vi "ETMF_ACP.vi"() -> ()   [LabVIEW 2019]
uses:
  <vilib>/Utility/error.llb/DialogType.ctl
  <vilib>/DAQmx/write.llb/DAQmx Write (Digital Bool 1Line 1Point).vi
  <vilib>/DAQmx/write.llb/DAQmx Write (Counter Frequency 1Chan 1Samp).vi
  <vilib>/DAQmx/miscellaneous.llb/DAQmx Fill In Error Info.vi
  <vilib>/DAQmx/create/channels.llb/DAQmx Create Channel (CO-Pulse Generation-Frequency).vi
  <vilib>/DAQmx/configure/timing.llb/DAQmx Timing (Implicit).vi
  <vilib>/addons/control/pid/pid.llb/PID (DBL).vi
  <vilib>/Utility/file.llb/Write Delimited Spreadsheet (string).vi
  <instrlib>/Agilent 34970/Agilent 34970.lvlib
  <resource>/objmgr/daqmx.rc
  <vilib>/addons/control/pid/NI_PID_pid.lvlib
  <instrlib>/Yokogawa WT200 Series/Yokogawa WT200 Series.lvlib
  <instrlib>/Agilent 681x Series/Agilent 681x Series.lvlib
panel:
  in  "Tab Control":T1(tab)
  in  "Ts":dbl=1.0
  out "Time":dbl=300.0 format="%<%H:%M:%S>t"
  in  "STOP":bool
  in  "Idenfier_Estufa":string="medsForno"
  in  "Estufa_ON":bool=TRUE
  in  "Frequency":dbl=1.0 format="%.6f"
  in  "PID gains":T2={"proportional gain (Kc)"=39.6, "integral time (Ti, min)"=14.617, "derivative time (Td, min)"=0.0} {"derivative time (Td, min)" format="%.3f"; "integral time (Ti, min)" format="%.3f"; "proportional gain (Kc)" format="%.6f"}
  out "Process variable and Setpoint":cluster{"initial PV":dbl, "SP:":dbl}(graph)
  out "MV":dbl(graph)
  in  "SP:":dbl(slide)=70.0 min=0.0 max=0.0 scale=25.0..70.0
  out "Temperature CH9 [degC]":dbl
  out "Temperature CH4 [degC]":dbl
  out "Iteration":i32
  out "Duty Cycle":sgl=0.1 min=0.1 max=99.9 format="%#_6f"
  out "PV":dbl
  in  "Tempo de integração (s)":u32=5 min=1 max=60 step=1
  out "Chart tensão numeric":cluster{"V(A)":dbl, "V(B)":dbl, "V(E)":dbl}(graph)={"V(A)"=0.0, "V(B)"=0.0, "V(E)"=228.25999450683594}
  out "Chart corrente numeric":cluster{"I(A)":dbl, "I(B)":dbl, "I(E)":dbl}(graph)={"I(A)"=0.0, "I(B)"=0.0, "I(E)"=0.14239999651908875}
  out "Chart potencia numeric":T3(graph)={"PC(A)"=0.0, "PC(B)"=7.200000254670158e-05, "PC(T)"=7.200000254670158e-05, "PL(A)"=0.0, "PL(B)"=0.0, "PL(T)"=0.0, "PC(E)"=1.0970638990402222, "PL(E)"=1.0099999904632568}
  in  "Realiza medição WT230":bool=TRUE
  in  "Medição contínua? WT230":bool=TRUE
  in  "Parâmetros serial":T4={"Serial VCC"="COM7", "timeout"=2, "baud rate"=600, "flow control"=0, "data bits"=8, "parity"=enum."None", "stop bits"=10, "termination char"=FALSE} {"stop bits" items=["1.0"=10, "1.5"=15, "2.0"=20]; "flow control" items=["None", "XON/XOFF", "RTS/CTS", "XON/XOFF & RTS/CTS", "DTR/DSR", "XON/XOFF & DTR/DSR"]}
  in  "Velocidade (RPM)":u16 min=1000 max=10000 step=100
  in  "Mensagem":T5(ring)=enum."Read power"
  in  "Limite de corrente":dbl min=0.0 max=0.4 step=0.01 format="%.4f"
  in  "Limite de tensão":dbl=30.0 min=0.0 max=30.0 step=0.5 format="%.4f"
  in  "Seta carga":bool
  in  "Enviar velocidade":bool
  in  "Envia mensagem":bool
  in  "Parar motor":bool
  out "Tradução":string
  out "Resposta":string
  in  "Liga Fonte":bool
  out "watt num cluster":T6
  out "Corrente de saída":dbl format="%.4f"
  out "Tensão de saída":dbl format="%.4f"
  out "t":dbl
  out "PL(T)":dbl
  out "PC(T)":dbl
  out "PC(E)":dbl
  out "PL(E)":dbl
  in  "Identifier_Watt":string="medsWatt"
  in  "Idenfier_Freio":string="medsFreio"
  in  "Manual":bool
  out "MV_I":dbl(graph)
  in  "PID gains MF":T2={"proportional gain (Kc)"=307.5977, "integral time (Ti, min)"=0.2636, "derivative time (Td, min)"=0.0} {"derivative time (Td, min)" format="%.3f"; "integral time (Ti, min)" format="%.3f"; "proportional gain (Kc)" format="%.6f"}
  out "Grafico MF ENS":cluster{"initial PV":dbl, "SP:":dbl}(graph)
  out "MV_MF":sgl=0.1 min=0.1 max=99.9 format="%#_6f"
  out "PV_MF":dbl
  in  "Ts MF":dbl=5.0
  in  "Automatic":bool
  in  "SP_MF":dbl(slide)=70.0 caption="SP:" min=0.0 max=0.0 scale=25.0..70.0
  in  "Ident_EnsTerMF":string="medsETMF"
  in  "Tab Control 2":enum32{"1-7", "8-15"}(tab)
  out "G. TP 1":cluster{dbl, "index":i32}(graph)
  out "TP 1":dbl
  out "TP 2":dbl
  out "G. TP 2":cluster{dbl, "index":i32}(graph)
  out "G. TP 3":cluster{dbl, "index":i32}(graph)
  out "TP 3":dbl
  out "G. TP 5":cluster{dbl, "index":i32}(graph)
  out "TP 5":dbl
  out "G. TP 6":cluster{dbl, "index":i32}(graph)
  out "TP 6":dbl
  out "G. TP 7":cluster{dbl, "index":i32}(graph)
  out "TP 7":dbl
  out "G. TP 8":cluster{dbl, "index":i32}(graph)
  out "TP 8":dbl
  out "G. TP 10":cluster{dbl, "index":i32}(graph)
  out "TP 10":dbl
  out "G. TP 11":cluster{dbl, "index":i32}(graph)
  out "TP 11":dbl
  out "G. TP 12":cluster{dbl, "index":i32}(graph)
  out "TP 12":dbl
  out "G. TP 13":cluster{dbl, "index":i32}(graph)
  out "TP 13":dbl
  out "G. TP 15":cluster{dbl, "index":i32}(graph)
  out "TP 15":dbl
  in  "Idenfier_Ens. Term.":string="medsETMA"
  out "Chart Temperatura":cluster{dbl, dbl, dbl, dbl, dbl, dbl}(graph)={21.505, 22.941, 24.092, 23.94, 23.972, 20.648}
  out "temperature num cluster":T7
  in  "Pulse Characteristic Value (%)":dbl=100.0 format="%#.4g"
  in  "Pulse Count":dbl=1.0 format="%#.4g"
  in  "Pulse Characteristic (0: Duty Cycle)":u16(ring) items=["Duty Cycle", "Pulse Width"]
  in  "Period (s)":dbl=10.0 format="%#.4g"
  in  "Output Frequency (60 Hz)":dbl=60.0 format="%#.4g"
  in  "Voltage Mode (0: Fix)":u16(ring) items=["Fixed", "Step", "Pulse", "List"]
  in  "Voltage Amplitude (1.0 V)":dbl=1.0 format="%#.4g"
  in  "Trigger Delay (s)":dbl=10.0 format="%#.5g"
  in  "Triggered Voltage Amplitude (V)":dbl=1.0 format="%#.4g"
  in  "Output Waveform Type (0: Sinusoid)":u16(ring) items=["Sinusoid", "Square", "Clipped Sinusoid", "User Specified"]
  in  "Peak Current Limit (13 A)":dbl=13.0 format="%#.4g"
  in  "RMS Current Limit (1 A)":dbl=1.0 format="%#.4g"
  in  "VISA resource name":refnum<visa-resource-name>
  out "CurMeas":T8
  out "PwrMeas":T9
  out "ACP_CUR":T10(graph)
  in  "Idenfier_Meas6812B":string="meds6812B"
  out "error out":errorcluster
  in  "Serial Configuration":T11={"Baud Rate"=9600, "Parity"=0, "Data Bits"=8} {"Data Bits" items=["7"=7, "8"=8]; "Parity" items=["None", "Odd", "Even", "Mark", "Space"]; "Baud Rate" items=["300"=300, "600"=600, "1200"=1200, "2400"=2400, "4800"=4800, "9600"=9600]}
  out "ACP_PWR":T12(graph)
  # "Controle de Temperatura da Estufa"
  # "Geral"
  # "Respostas do Sistema em Malha Fechada"
  # "Controles"
  # "Medidas"
  # "Freio"
  # "Wattímetro WT230 Yokogawa"
  # "Controles:"
  # "Controles"
  # "Medidas"
  # "Respostas temporais"
  # "Medidas"
  # "Inversor de Frequência"
  # "Controles"
  # "Comandos"
  # "Parâmetros Serial"
  # "Controle Automático do Ensaio de Estresse Térmico"
  # "Geral"
  # "Controles"
  # "Medidas"
  # "Temperaturas dos Termopares"
  # "Nome do arquivo:"
  # "Legenda:"
  # "TP 1: Termopar do Capacitor C011"
  # "TP 3: Termopar do Choke L001"
  # "TP 2: Termopar do Capacitor C009"
  # "TP 5: Termopar do Capacitor C006"
  # "TP 6: Termopar do Fusível F002"
  # "TP 7: Termopar do Conector CN204"
  # "TP 8: Termopar do CI SMPS IC 100"
  # "TP 10: Termopar do Indutor L100"
  # "TP 11: Termopar do Capacitor C112"
  # "TP 12: Termopar do Capacitor C504"
  # "TP 13: Termopar do Microcontrolador IC601"
  # "TP 15: Termopar do Dissipador"
  # "Temperaturas do Motor/Freio"
  # "Gráficos:"
  # "Configurações da Saída"
  # "Potências:"
  # "Trigger"
  # "Forma de Onda"
  # "Correntes:"
  # "Proteção contra Sobrecorrente"
  # "Comunicação"
  # "Fonte AC Programável - Agilent 6812B"
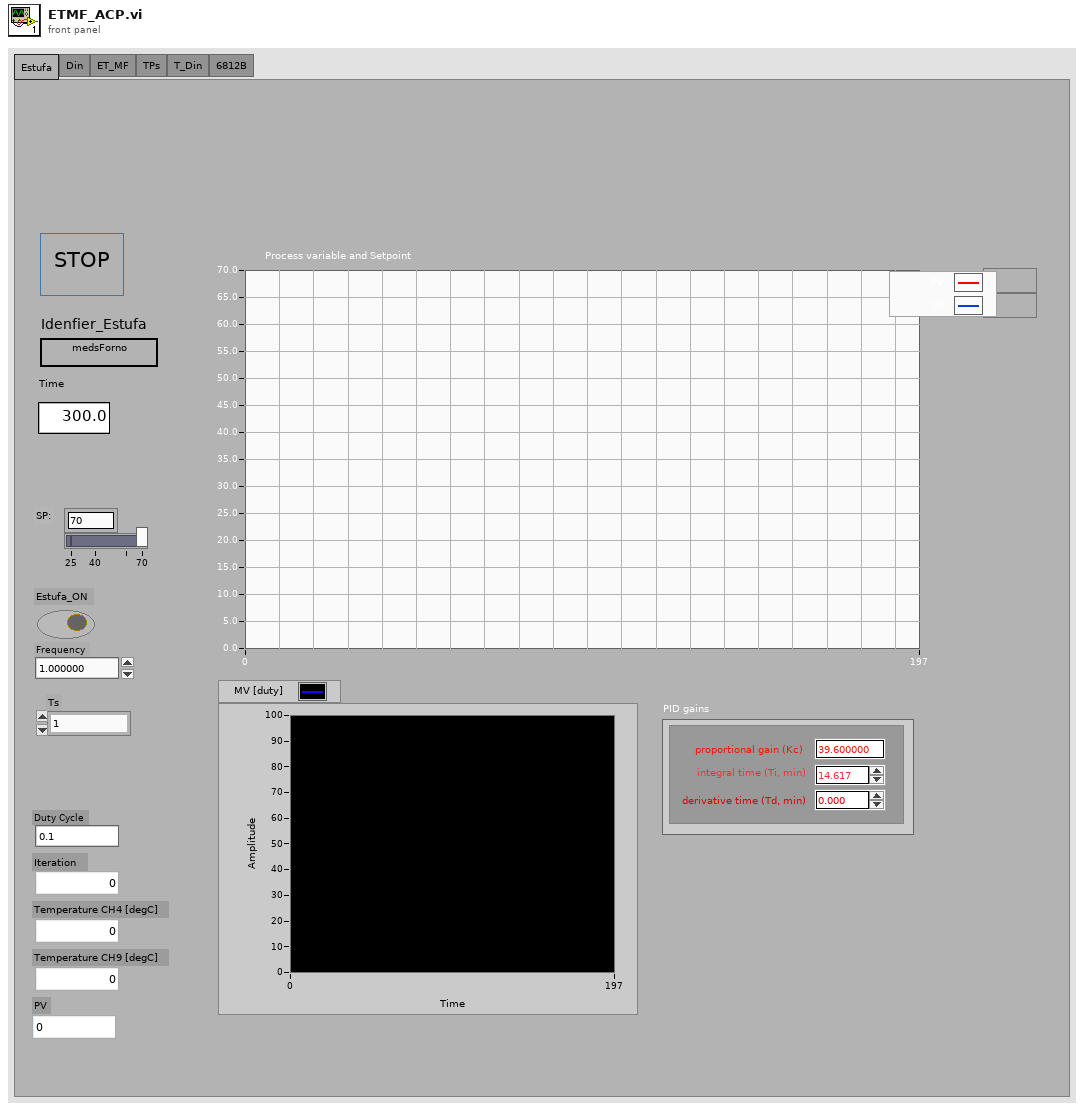
[diagram p1: front panel]
types:
  T1 = enum32{"Estufa", "Din", "ET_MF", "TPs", "T_Din", "6812B"}
  T2 = cluster{"proportional gain (Kc)":dbl, "integral time (Ti, min)":dbl, "derivative time (Td, min)":dbl}
  T3 = cluster{"PC(A)":dbl, "PC(B)":dbl, "PC(T)":dbl, "PL(A)":dbl, "PL(B)":dbl, "PL(T)":dbl, "PC(E)":dbl, "PL(E)":dbl}
  T4 = cluster{"Serial VCC":refnum<visa-resource-name>, "timeout":u32, "baud rate":u32, "flow control":u16, "data bits":u16, "parity":enum16{"None", "Odd", "Even", "Mark", "Space"}, "stop bits":u16, "termination char":bool}
  T5 = enum16{"Read set speed", "Read operation status", "Read power", "Read starting trials", "Read bus voltage", "Read temperature", "Read power limitation", "Read PWM mode", "Read PWM frequency", "Read real speed"}
  T6 = cluster{"V(A)":dbl, "I(A)":dbl, "V(B)":dbl, "I(B)":dbl, "PC(A)":dbl, "PC(B)":dbl, "PC(T)":dbl, "PL(T)":dbl, "PL(B)":dbl, "PL(A)":dbl, "V(E)":dbl, "PL(E)":dbl, "PC(E)":dbl, "I(E)":dbl, "t":dbl}
  T7 = cluster{"t1 freio":dbl, "t2 bobina":dbl, "t5 bobina":dbl, "t4 estator":dbl, "t3 estator":dbl, "t6 amb":dbl}
  T8 = cluster{"Peak Current":dbl, "DC Current":dbl, "AC RMS Current":dbl, "AC + DC RMS Cur":dbl}
  T9 = cluster{"Power Factor":dbl, "Reactive Power":dbl, "DC Power":dbl, "Real Power":dbl, "Apparent Power":dbl, "Total Power":dbl}
  T10 = cluster{"Peak Current":dbl, "AC RMS Current":dbl, "AC + DC RMS Current":dbl}
  T11 = cluster{"Baud Rate":u32, "Parity":u16, "Data Bits":u16}
  T12 = cluster{"Reactive Power":dbl, "Apparent Power":dbl, "Total Power":dbl}
  T13 = enum16{"Start Comm.", "End Comm.", "Wait", "Send Static Message", "Set Speed"}
  T14 = enum16{"Thermocouple", "Thermistor", "RTD", "4-Wire RTD", "Default (Last)"}
  T15 = enum8{"Enabled", "Disabled", "Disabled and Grayed Out"}
  T16 = cluster{"Peak Current":dbl, "DC Current":dbl, "AC RMS Current":dbl, "AC + DC RMS Current":dbl}
  T17 = cluster{"Peak Current":dbl, "AC RMS Current":dbl, "AC + DC RMS Cur":dbl}
  T18 = typedef "DialogType.ctl" = u16
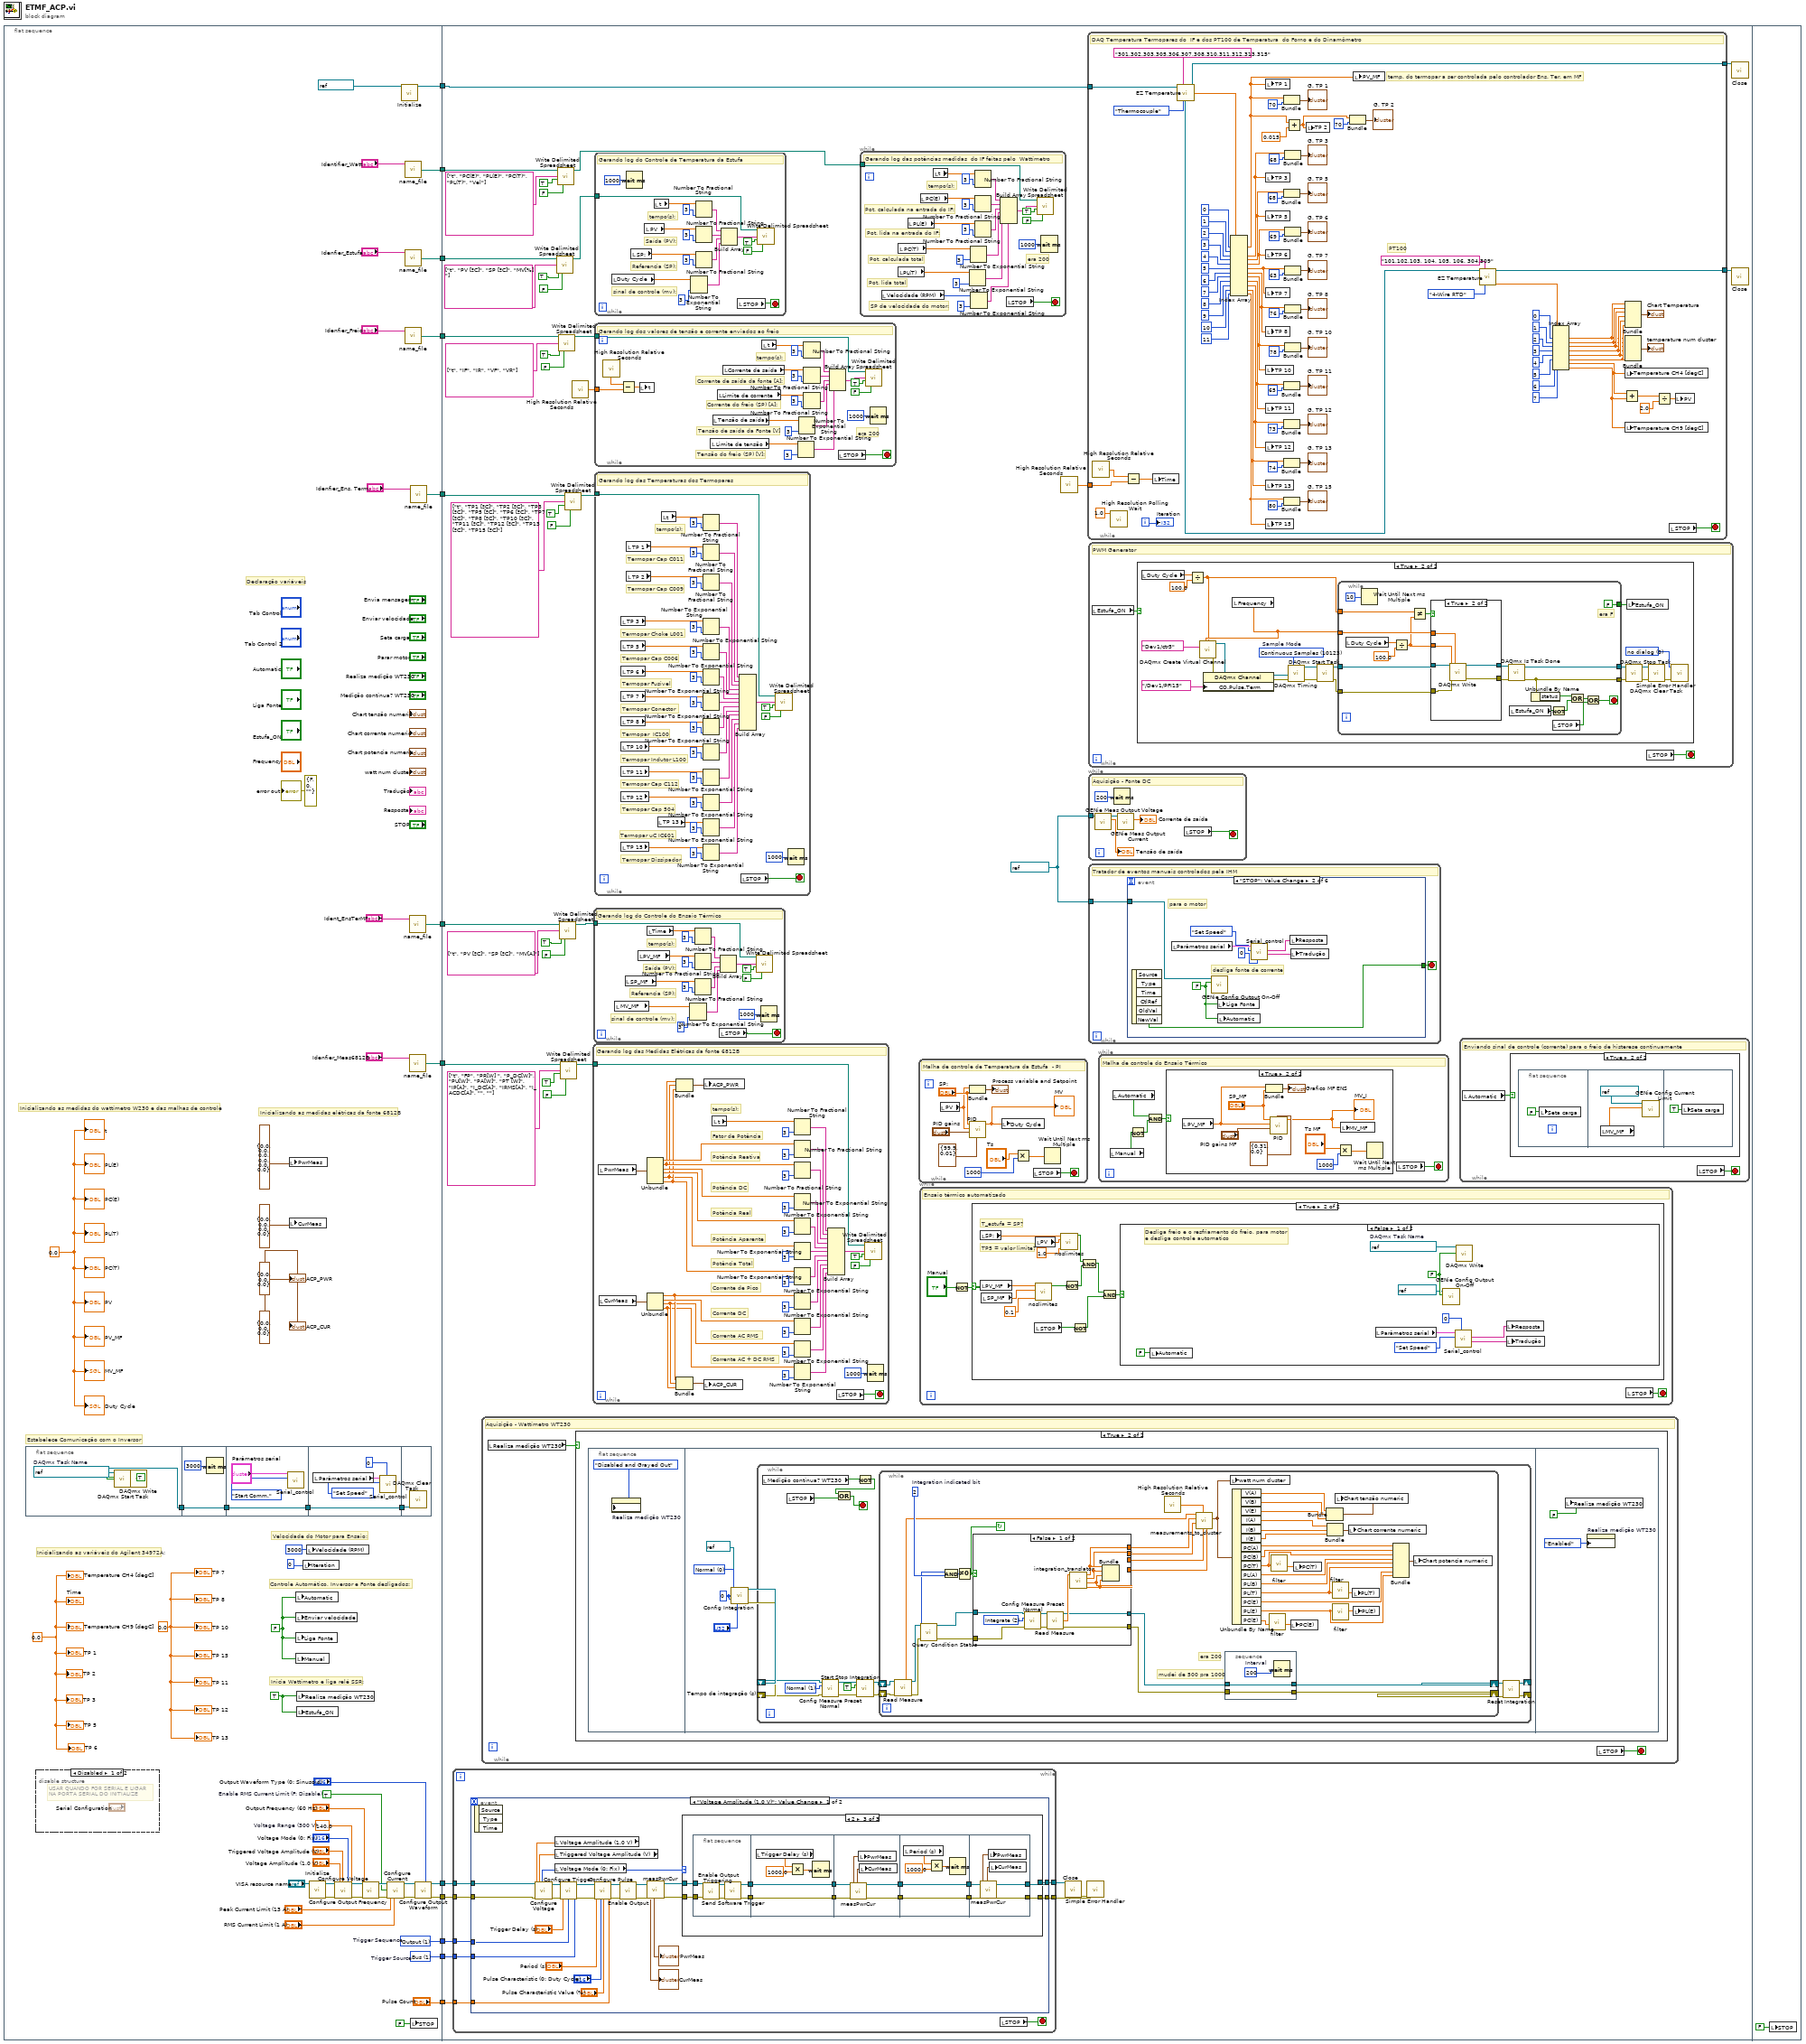
[diagram p0: block diagram]
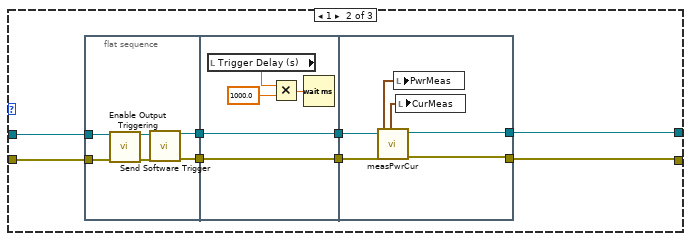
[diagram p4: hidden frame]
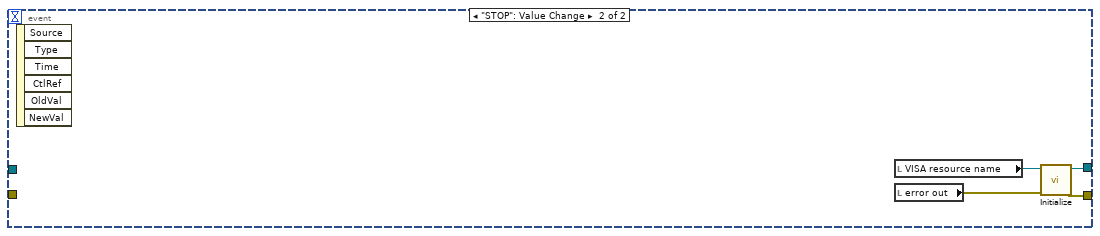
[diagram p5: hidden frame]
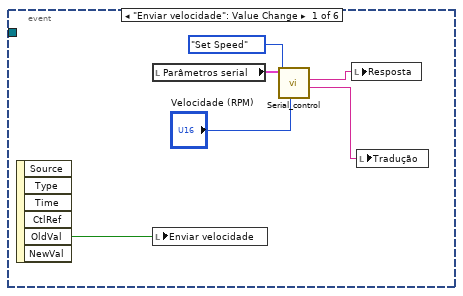
[diagram p7: hidden frame]
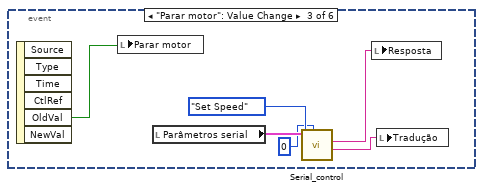
[diagram p8: hidden frame]
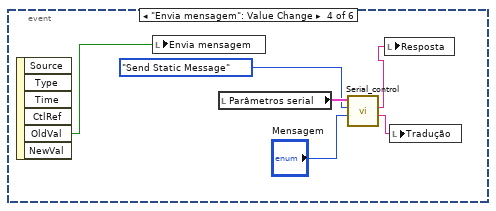
[diagram p9: hidden frame]
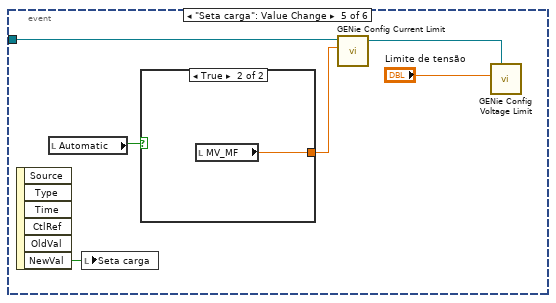
[diagram p10: hidden frame]
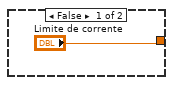
[diagram p11: hidden frame]
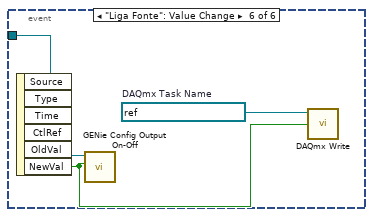
[diagram p12: hidden frame]
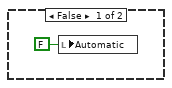
[diagram p14: hidden frame]
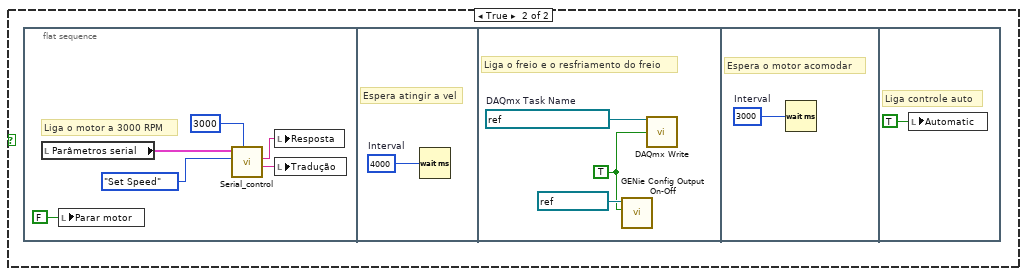
[diagram p15: hidden frame]
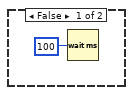
[diagram p16: hidden frame]
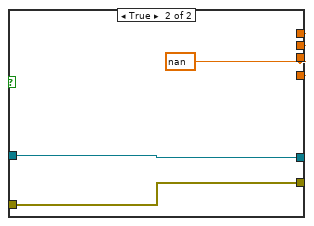
[diagram p17: hidden frame]
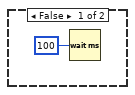
[diagram p18: hidden frame]
diagram:
  n1 = flat-sequence {
    tunnel: [w64] -> w12
    tunnel: [w63] -> w11
    tunnel: [w59] -> w10
    tunnel: [w57] -> w9
    tunnel: [w55] -> w8
    tunnel: [w52] -> w7
    tunnel: [w48] -> w6
    tunnel: [w25] -> w5
    tunnel: [w24] -> w4
    tunnel: [w22] -> w3
    tunnel: [w23] -> w2
    tunnel: ["Pulse Count"] -> w1
    tunnel: w12 -> [w98]
    tunnel: w11 -> [w118]
    tunnel: w10 -> [w117]
    tunnel: w9 -> [w112]
    tunnel: w8 -> [w103]
    tunnel: w7 -> [w94]
    tunnel: w6 -> [w91]
    tunnel: w5 -> [w84]
    tunnel: w4 -> [w83]
    tunnel: w3 -> [w82]
    tunnel: w2 -> [w81]
    tunnel: w1 -> [w80]
    frame #0 {
      w23 = 1 items=["Immediate", "Bus", "External", "Phase", "Trigger Out"]  # Trigger Source
      w22 = 1 items=["Output"=1, "Synchronous Source"=2, "Measurement"=3]  # Trigger Sequence
      w27 = TRUE  # Enable RMS Current Limit (F: Disable)
      w26 = 140.0  # Voltage Range (300 V)
      w45 = 0.0 ("Temperature 1")
      w46 = 0.0 ("PC(E)")
      w49 = FALSE ("Automatic")
      w50 = TRUE ("Realiza medição WT230")
      w54 = 0.0 ("Temperature 1")
      # "Estabelece Comunicação com o Inversor"
      # "Inicializando as variáveis do Agilent 34972A:"
      # "Inicializando as medidas do wattímetro W230 e das malhas de controle"
      # "Inicializando as medidas elétricas da fonte 6812B"
      # "Inicia Wattímetro e liga relé SSR:"
      # "Controle Automático, Inversor e Fonte desligados:"
      # "Velocidade do Motor para Ensaio:"
      # "Declaração variáveis"
      n2 = flat-sequence {
        tunnel: [w66] -> w16
        tunnel: w16 -> [w69]
        tunnel: [w69] -> w15
        tunnel: w15 -> [w71]
        tunnel: [w71] -> w14
        tunnel: w14 -> [w74]
        tunnel: [w74] -> w13
        tunnel: w13 -> [w78]
        frame #0 {
          w67 = refnum<k21> "alimentacao_inversor"  # DAQmx Task Name
          n3 = call <vilib>:"DAQmx Start Task.vi"("task/channels in"=w67) -> ("task out"=w66:refnum<k21>)  [unwired: 13 in, 1 out]
          n4 = call-poly <vilib>:"DAQmx Write.vi"("task/channels in"=w66, "data"=TRUE) -> ()  [unwired: 11 in, 3 out]
        }
        frame #1 {
          n5 = Wait (ms)(milliseconds to wait=u32 3000) -> ()  [unwired: 1 out]
        }
        frame #2 {
          n6 = call "Serial_control.vi"("Função"=T13."Start Comm.", "comm cluster"="Parâmetros serial") -> ()  [unwired: 3 in, 4 out]
        }
        frame #3 {
          n7 = local read "Parâmetros serial"() -> (w76:T4)
          n8 = call "Serial_control.vi"("Enviar número"=u16 0, "Função"=T13."Set Speed", "comm cluster"=w76) -> ()  [unwired: 2 in, 4 out]
        }
        frame #4 {
          n9 = call <vilib>:"DAQmx Clear Task.vi"("task in"=w78) -> ()  [unwired: 14 in, 1 out]
        }
      }
      n10 = disable-structure shown="Disabled" {
        frame Disabled {
          # "USAR QUANDO FOR SERIAL E LIGAR \nNA PORTA SERIAL DO INITIALIZE"
        }
        frame Enabled {
        }
      }
      n11 = local write "PwrMeas"(T9 {"Power Factor"=0.0, "Reactive Power"=0.0, "DC Power"=0.0, "Real Power"=0.0, "Apparent Power"=0.0, "Total Power"=0.0} ("PwrMeas")) -> ()
      n12 = local write "CurMeas"(T8 {"Peak Current"=0.0, "DC Current"=0.0, "AC RMS Current"=0.0, "AC + DC RMS Cur"=0.0} ("CurMeas")) -> ()
      n13 = local write "Automatic"(w49) -> ()
      n14 = local write "Enviar velocidade"(w49) -> ()
      n15 = local write "Liga Fonte"(w49) -> ()
      n16 = local write "Manual"(w49) -> ()
      n17 = local write "Realiza medição WT230"(w50) -> ()
      n18 = local write "Estufa_ON"(w50) -> ()
      n19 = local write "Iteration"(0 ("Iteration")) -> ()
      n20 = local write "Velocidade (RPM)"(u16 3000 ("Velocidade (RPM)")) -> ()
      n21 = call <instrlib>:"Initialize.vi"("VISA resource name"="VISA resource name") -> ("error out"=w39:errorcluster)  [unwired: 9 in, 1 out]
      n22 = call <instrlib>:"Configure Voltage.vi"("VISA resource name"="VISA resource name", "Triggered Voltage Amplitude (1.0 V)"="Triggered Voltage Amplitude (V)", "Voltage Range (300 V)"=w26, "Voltage Amplitude (1.0 V)"="Voltage Amplitude (1.0 V)", "Voltage Mode (0: Fix)"="Voltage Mode (0: Fix)", "error in (no error)"=w39) -> ("VISA resource name out"=w31:refnum<visa-resource-name>, "error out"=w30:errorcluster)  [unwired: 8 in]
      n23 = call <instrlib>:"Configure Output Frequency.vi"("VISA resource name"=w31, "Output Frequency (60 Hz)"="Output Frequency (60 Hz)", "error in (no error)"=w30) -> ("VISA resource name out"=w41:refnum<visa-resource-name>, "error out"=w42:errorcluster)  [unwired: 11 in]
      n24 = call <instrlib>:"Configure Current.vi"("VISA resource name"=w41, "Enable RMS Current Limit (F: Disable)"=w27, "RMS Current Limit (1 A)"="RMS Current Limit (1 A)", "error in (no error)"=w42, "Peak Current Limit (13 A)"="Peak Current Limit (13 A)") -> ("VISA resource name out"=w29:refnum<visa-resource-name>, "error out"=w28:errorcluster)  [unwired: 9 in]
      n25 = call <instrlib>:"Initialize.vi"("VISA Resource Name"=refnum<visa-resource-name> "Agilent" ("VISA AGILENT")) -> ("VISA Resource Name Out"=w64:refnum<visa-resource-name>)  [unwired: 13 in, 1 out]
      n26 = call "name_file.vi"("Identifier"="Identifier_Watt") -> ("appended path"=w59:path)  [unwired: 2 in]
      n27 = call "name_file.vi"("Identifier"="Idenfier_Estufa") -> ("appended path"=w63:path)  [unwired: 2 in]
      n28 = call "name_file.vi"("Identifier"="Idenfier_Freio") -> ("appended path"=w57:path)  [unwired: 2 in]
      n29 = call "name_file.vi"("Identifier"="Ident_EnsTerMF") -> ("appended path"=w52:path)  [unwired: 2 in]
      n30 = call "name_file.vi"("Identifier"="Idenfier_Meas6812B") -> ("appended path"=w48:path)  [unwired: 2 in]
      n31 = call "name_file.vi"("Identifier"="Idenfier_Ens. Term.") -> ("appended path"=w55:path)  [unwired: 2 in]
      n32 = local write "STOP"(FALSE ("STOP")) -> ()
      n33 = call <instrlib>:"Configure Output Waveform.vi"("VISA resource name"=w29, "Output Waveform Type (0: Sinusoid)"="Output Waveform Type (0: Sinusoid)", "error in (no error)"=w28) -> ("VISA resource name out"=w25:refnum<visa-resource-name>, "error out"=w24:errorcluster)  [unwired: 11 in]
      "Temperature CH4 [degC]" <- w54
      "Temperature CH9 [degC]" <- w54
      "Time" <- w54
      "Duty Cycle" <- w46
      "PV" <- w46
      "PC(T)" <- w46
      "PL(T)" <- w46
      "PC(E)" <- w46
      "t" <- w46
      "PL(E)" <- w46
      "TP 1" <- w54
      "TP 2" <- w54
      "TP 3" <- w54
      "TP 5" <- w54
      "TP 6" <- w54
      "TP 7" <- w45
      "TP 8" <- w45
      "TP 10" <- w45
      "TP 11" <- w45
      "TP 12" <- w45
      "TP 13" <- w45
      "TP 15" <- w45
      "MV_MF" <- w46
      "PV_MF" <- w46
      "error out" <- errorcluster {"status"=FALSE, "code"=0, "source"=""} ("error out")
      "ACP_CUR" <- T10 {"Peak Current"=0.0, "AC RMS Current"=0.0, "AC + DC RMS Current"=0.0} ("ACP_CUR")
      "ACP_PWR" <- T12 {"Reactive Power"=0.0, "Apparent Power"=0.0, "Total Power"=0.0} ("ACP_PWR")
    }
    frame #1 {
      w92 = refnum<visa-resource-name> "Lambda" ("VISA name")
      n34 = while {
        tunnel: w84 -> [w130]
        tunnel: w83 -> [w129]
        tunnel: [w123] -> w86
        tunnel: [w124] -> w85
        tunnel: w81 -> [w127]
        tunnel: w82 -> [w126]
        tunnel: w80 -> [w125]
        stop <- w128 stop-if-true
        n35 = event shown="[0] \"Voltage Amplitude (1.0 V)\": Value Change" {
          selector: _ -> [_ _]
          dyn-events: _ -> [_ _]
          timeout: _ -> [_ _]
          tunnel: w130 -> [w154 _]
          tunnel: w129 -> [w153 _]
          tunnel: w127 -> [w143 _]
          tunnel: w126 -> [w142 _]
          tunnel: w125 -> [w137 _]
          tunnel: [w135 w225] -> w124
          tunnel: [w134 w226] -> w123
          event "Voltage Amplitude (1.0 V)": Value Change {
            n36 = event-data() -> ()  [unwired: 1 in, 3 out]
            n37 = local read "Voltage Amplitude (1.0 V)"() -> (w152:dbl)
            n38 = local read "Triggered Voltage Amplitude (V)"() -> (w136:dbl)
            n39 = local read "Voltage Mode (0: Fix)"() -> (w133:u16)
            n40 = call <instrlib>:"Configure Voltage.vi"("VISA resource name"=w154, "Triggered Voltage Amplitude (1.0 V)"=w136, "Voltage Amplitude (1.0 V)"=w152, "Voltage Mode (0: Fix)"=w133, "error in (no error)"=w153) -> ("VISA resource name out"=w149:refnum<visa-resource-name>, "error out"=w148:errorcluster)  [unwired: 9 in]
            n41 = call <instrlib>:"Configure Trigger.vi"("VISA resource name"=w149, "Trigger Sequence (1: Output 1)"=w143, "Trigger Source (0: Immediate)"=w142, "error in (no error)"=w148, "Trigger Delay (0 s)"="Trigger Delay (s)") -> ("VISA resource name out"=w150:refnum<visa-resource-name>, "error out"=w151:errorcluster)  [unwired: 9 in]
            n42 = call <instrlib>:"Configure Pulse.vi"("VISA resource name"=w150, "Pulse Count (1)"=w137, "Period (0.0333 s)"="Period (s)", "error in (no error)"=w151, "Pulse Characteristic (0: Duty Cycle)"="Pulse Characteristic (0: Duty Cycle)", "Pulse Characteristic Value (50)"="Pulse Characteristic Value (%)") -> ("VISA resource name out"=w147:refnum<visa-resource-name>, "error out"=w146:errorcluster)  [unwired: 8 in]
            n43 = call <instrlib>:"Enable Output.vi"("VISA resource name"=w147, "error in (no error)"=w146) -> ("VISA resource name out"=w156:refnum<visa-resource-name>, "error out"=w155:errorcluster)  [unwired: 12 in]
            n44 = call "measPwrCur.vi"("VISA resource name"=w156, "error in (no error)"=w155) -> ("PwrMeas"=→"PwrMeas":T9, "CurMeas"=→"CurMeas":T16, "VISA resource name out"=w145:refnum<visa-resource-name>, "error out"=w144:errorcluster)  [unwired: 3 in]
            n45 = case shown="2" w133 {
              tunnel: w145 -> [w158 w166 w189]
              tunnel: w144 -> [w157 w165 w188]
              tunnel: [w157 w160 w184] -> w135
              tunnel: [w158 w159 w185] -> w134
              frame 0, Default {
              }
              frame 1 {
                n46 = flat-sequence {
                  tunnel: w166 -> [w170]
                  tunnel: w165 -> [w169]
                  tunnel: [w168] -> w163
                  tunnel: [w167] -> w161
                  tunnel: [w177] -> w164
                  tunnel: w163 -> [w177]
                  tunnel: [w176] -> w162
                  tunnel: w161 -> [w176]
                  tunnel: w164 -> [w181]
                  tunnel: w162 -> [w178]
                  tunnel: [w179] -> w160
                  tunnel: [w180] -> w159
                  frame #0 {
                    n47 = call <instrlib>:"Enable Output Triggering.vi"("VISA resource name"=w170, "error in (no error)"=w169) -> ("VISA resource name out"=w171:refnum<visa-resource-name>, "error out"=w172:errorcluster)  [unwired: 12 in]
                    n48 = call <instrlib>:"Send Software Trigger.vi"("VISA resource name"=w171, "error in (no error)"=w172) -> ("VISA resource name out"=w168:refnum<visa-resource-name>, "error out"=w167:errorcluster)  [unwired: 12 in]
                  }
                  frame #1 {
                    n49 = local read "Trigger Delay (s)"() -> (w175:dbl)
                    n50 = Multiply(x=w175, y=1000.0) -> (x*y=w173:dbl)
                    n51 = Wait (ms)(milliseconds to wait=w173) -> ()  [unwired: 1 out]
                  }
                  frame #2 {
                    n52 = call "measPwrCur.vi"("VISA resource name"=w181, "error in (no error)"=w178) -> ("PwrMeas"=w182:T9, "CurMeas"=w183:T16, "VISA resource name out"=w180:refnum<visa-resource-name>, "error out"=w179:errorcluster)  [unwired: 3 in]
                    n53 = local write "PwrMeas"(w182) -> ()
                    n54 = local write "CurMeas"(w183) -> ()
                  }
                }
              }
              frame 2 {
                n55 = flat-sequence {
                  tunnel: [w199] -> w195
                  tunnel: [w198] -> w194
                  tunnel: w189 -> [w197]
                  tunnel: w188 -> [w196]
                  tunnel: [w206] -> w193
                  tunnel: w195 -> [w206]
                  tunnel: [w205] -> w192
                  tunnel: w194 -> [w205]
                  tunnel: w193 -> [w212]
                  tunnel: w192 -> [w211]
                  tunnel: [w210] -> w191
                  tunnel: [w209] -> w190
                  tunnel: w191 -> [w213]
                  tunnel: w190 -> [w214]
                  tunnel: [w214] -> w187
                  tunnel: [w213] -> w186
                  tunnel: w187 -> [w222]
                  tunnel: w186 -> [w221]
                  tunnel: [w220] -> w185
                  tunnel: [w219] -> w184
                  frame #0 {
                    n56 = call <instrlib>:"Enable Output Triggering.vi"("VISA resource name"=w197, "error in (no error)"=w196) -> ("VISA resource name out"=w200:refnum<visa-resource-name>, "error out"=w201:errorcluster)  [unwired: 12 in]
                    n57 = call <instrlib>:"Send Software Trigger.vi"("VISA resource name"=w200, "error in (no error)"=w201) -> ("VISA resource name out"=w199:refnum<visa-resource-name>, "error out"=w198:errorcluster)  [unwired: 12 in]
                  }
                  frame #1 {
                    n58 = local read "Trigger Delay (s)"() -> (w204:dbl)
                    n59 = Multiply(x=w204, y=1000.0) -> (x*y=w202:dbl)
                    n60 = Wait (ms)(milliseconds to wait=w202) -> ()  [unwired: 1 out]
                  }
                  frame #2 {
                    n61 = call "measPwrCur.vi"("VISA resource name"=w212, "error in (no error)"=w211) -> ("PwrMeas"=w207:T9, "CurMeas"=w208:T16, "VISA resource name out"=w209:refnum<visa-resource-name>, "error out"=w210:errorcluster)  [unwired: 3 in]
                    n62 = local write "PwrMeas"(w207) -> ()
                    n63 = local write "CurMeas"(w208) -> ()
                  }
                  frame #3 {
                    n64 = local read "Period (s)"() -> (w215:dbl)
                    n65 = Multiply(x=w215, y=1000.0) -> (x*y=w217:dbl)
                    n66 = Wait (ms)(milliseconds to wait=w217) -> ()  [unwired: 1 out]
                  }
                  frame #4 {
                    n67 = call "measPwrCur.vi"("VISA resource name"=w222, "error in (no error)"=w221) -> ("PwrMeas"=w223:T9, "CurMeas"=w218:T16, "VISA resource name out"=w220:refnum<visa-resource-name>, "error out"=w219:errorcluster)  [unwired: 3 in]
                    n68 = local write "PwrMeas"(w223) -> ()
                    n69 = local write "CurMeas"(w218) -> ()
                  }
                }
              }
            }
          }
          event "STOP": Value Change {
            n70 = event-data() -> ()  [unwired: 1 in, 6 out]
            n71 = local read "VISA resource name"() -> (w227:refnum<visa-resource-name>)
            n72 = local read "error out"() -> (w224:errorcluster)
            n73 = call <instrlib>:"Initialize.vi"("error in (no error)"=w224, "VISA resource name"=w227) -> ("error out"=w225:errorcluster, "VISA resource name out"=w226:refnum<visa-resource-name>)  [unwired: 8 in]
          }
        }
        n74 = local read "STOP"() -> (w128:bool)
      }
      n75 = while {
        stop <- w570 stop-if-true
        # "Aquisição - Wattímetro WT230"
        n76 = local read "Realiza medição WT230"() -> (w571:bool)
        n77 = case shown="True" w571 {
          frame False {
            n78 = Wait (ms)(milliseconds to wait=u32 100) -> ()  [unwired: 1 out]
          }
          frame True {
            n79 = flat-sequence {
              frame #0 {
                n80 = property on="Realiza medição WT230" class="Bool (strict)"("DisabledEnum"=T15."Disabled and Grayed Out" ("Disabled")) -> ()  [unwired: 2 in, 2 out]
              }
              frame #1 {
                w576 = u16 0 items=["Normal", "Continuous"] ("Integ Mode (0: Normal)")
                w577 = u32 0 ("Hour (0)")
                n81 = call <instrlib>:"Config Integration.vi"("VISA resource name"=refnum<visa-resource-name> "WT", "Integ Mode (0: Normal)"=w576, "Hour (0)"=w577, "Minute (0)"=w577, "Second (0)"="Tempo de integração (s)") -> ("VISA resource name out"=w579:refnum<visa-resource-name>, "error out"=w578:errorcluster)  [unwired: 9 in]
                n82 = while {
                  shift-right: [w583] -> _
                  shift-left: w579 -> [w581]
                  shift-right: [w582] -> _
                  shift-left: w578 -> [w580]
                  stop <- w584 stop-if-true
                  w590 = u16 1 items=["Clear", "Normal", "Integrate"] ("Preset Pattern (0: Clear)")
                  n83 = local read "Medição contínua? WT230"() -> (w586:bool)
                  n84 = local read "STOP"() -> (w587:bool)
                  n85 = call <instrlib>:"Config Measure Preset Normal.vi"("VISA resource name"=w581, "Preset Pattern (0: Clear)"=w590, "error in (no error)"=w580) -> ("VISA resource name out"=w592:refnum<visa-resource-name>, "error out"=w591:errorcluster)  [unwired: 11 in]
                  n86 = call <instrlib>:"Start Stop Integration.vi"("VISA resource name"=w592, "Start/Stop (F: Stop)"=TRUE, "error in (no error)"=w591) -> ("VISA resource name out"=w595:refnum<visa-resource-name>, "error out"=w594:errorcluster)  [unwired: 11 in]
                  n87 = Not(x=w586) -> (.not. x?=w585:bool)
                  n88 = Or(x=w585, y=w587) -> (x .or. y?=w584:bool)
                  n89 = while {
                    shift-left: w595 -> [w635]
                    shift-right: [w623] -> w589
                    shift-left: w594 -> [w632]
                    shift-right: [w621] -> w588
                    stop <- w631 continue-if-true
                    w638 = u16 2  # Integration indicated bit
                    # "era 200"
                    # "mudei de 500 pra 1000"
                    n90 = call <instrlib>:"Read Measure.vi"("VISA resource name"=w635, "error in (no error)"=w632) -> ("VISA resource name out"=w634:refnum<visa-resource-name>, "Measure Value"=w625:sgl[], "error out"=w633:errorcluster)  [unwired: 10 in, 1 out]
                    n91 = call <instrlib>:"Query Condition Status.vi"("VISA resource name"=w634, "error in (no error)"=w633) -> ("VISA resource name out"=w620:refnum<visa-resource-name>, "Condition"=w636:u16, "error out"=w619:errorcluster)  [unwired: 11 in]
                    n92 = And(x=w636, y=w638) -> (x .and. y?=w637:u16)
                    n93 = Not Equal To 0?(x=w637) -> (x != 0?=w631:bool)
                    n94 = case shown="False" w631 {
                      tunnel: [w649 w656] -> w630
                      tunnel: [w648 w656] -> w629
                      tunnel: [w647 w656] -> w628
                      tunnel: [w646 w656] -> w627
                      tunnel: [w645 w655] -> w624
                      tunnel: [w644 w654] -> w622
                      tunnel: w620 -> [w643 w655]
                      tunnel: w619 -> [w642 w654]
                      frame False {
                        w650 = u16 2 items=["Clear", "Normal", "Integrate"] ("Preset Pattern (0: Clear)")
                        n95 = call <instrlib>:"Config Measure Preset Normal.vi"("VISA resource name"=w643, "Preset Pattern (0: Clear)"=w650, "error in (no error)"=w642) -> ("VISA resource name out"=w653:refnum<visa-resource-name>, "error out"=w652:errorcluster)  [unwired: 11 in]
                        n96 = call <instrlib>:"Read Measure.vi"("VISA resource name"=w653, "error in (no error)"=w652) -> ("VISA resource name out"=w645:refnum<visa-resource-name>, "Measure Value"=w651:sgl[], "error out"=w644:errorcluster)  [unwired: 10 in, 1 out]
                        n97 = call "integration_translator.vi"("Valores integração"=w651) -> ("PI(E)"=w646:sgl, "PI(T)"=w647:sgl, "PI(B)"=w648:sgl, "PI(A)"=w649:sgl)  [unwired: 7 in]
                        n98 = Bundle("PI(A)"=w649, "PI(B)"=w648, "PI(T)"=w647, "PI(E)"=w646) -> ()  [unwired: 1 in, 1 out]
                      }
                      frame True {
                        w656 = nan
                      }
                    }
                    n99 = call <vilib>:"High Resolution Relative Seconds.vi"() -> ("relative seconds"=w626:dbl)
                    n100 = call "measurements_to_cluster.vi"("PI(E)"=w627, "PI(T)"=w628, "relative seconds"=w626, "PI(B)"=w629, "PI(A)"=w630, "Measure Value"=w625) -> ("watt cluster"=w618:T6)  [unwired: 4 in, 1 out]
                    n101 = stacked-sequence {
                      tunnel: w624 -> [w640]
                      tunnel: [w640] -> w623
                      tunnel: w622 -> [w639]
                      tunnel: [w639] -> w621
                      frame #0 {
                        w641 = u32 200  # Interval
                        n102 = Wait (ms)(milliseconds to wait=w641) -> ()  [unwired: 1 out]
                      }
                    }
                    n103 = local write "watt num cluster"(w618) -> ()
                    n104 = Unbundle By Name(w618) -> ("V(A)"=w613:dbl, "V(B)"=w612:dbl, "V(E)"=w611:dbl, "I(A)"=w610:dbl, "I(B)"=w609:dbl, "I(E)"=w608:dbl, "PC(A)"=w607:dbl, "PC(B)"=w606:dbl, "PC(T)"=w605:dbl, "PL(A)"=w603:dbl, "PL(B)"=w602:dbl, "PL(T)"=w601:dbl, "PC(E)"=w600:dbl, "PL(E)"=w599:dbl, "PC(E)"=w597:dbl)
                    n105 = call "filter.vi"("input"=w597) -> ("output"=w596:dbl)  [unwired: 10 in]
                    n106 = call "filter.vi"("input"=w605) -> ("output"=w604:dbl)  [unwired: 10 in]
                    n107 = local write "PC(E)"(w596) -> ()
                    n108 = local write "PC(T)"(w604) -> ()
                    n109 = Bundle("V(A)"=w613, "V(B)"=w612, "V(E)"=w611) -> (w617:cluster{"V(A)":dbl, "V(B)":dbl, "V(E)":dbl})  [unwired: 1 in]
                    n110 = Bundle("I(A)"=w610, "I(B)"=w609, "I(E)"=w608) -> (w616:cluster{"I(A)":dbl, "I(B)":dbl, "I(E)":dbl})  [unwired: 1 in]
                    n111 = call "filter.vi"("input"=w601) -> ("output"=w615:dbl)  [unwired: 10 in]
                    n112 = call "filter.vi"("input"=w599) -> ("output"=w614:dbl)  [unwired: 10 in]
                    n113 = local write "Chart tensão numeric"(w617) -> ()
                    n114 = local write "Chart corrente numeric"(w616) -> ()
                    n115 = local write "PL(T)"(w615) -> ()
                    n116 = local write "PL(E)"(w614) -> ()
                    n117 = Bundle("PC(A)"=w607, "PC(B)"=w606, "PC(T)"=w605, "PL(A)"=w603, "PL(B)"=w602, "PL(T)"=w601, "PC(E)"=w600, "PL(E)"=w599) -> (w598:T3)  [unwired: 1 in]
                    n118 = local write "Chart potencia numeric"(w598) -> ()
                  }
                  n119 = call <instrlib>:"Reset Integration.vi"("VISA resource name"=w589, "error in (no error)"=w588) -> ("VISA resource name out"=w583:refnum<visa-resource-name>, "error out"=w582:errorcluster)  [unwired: 12 in]
                }
              }
              frame #2 {
                n120 = local write "Realiza medição WT230"(FALSE ("Realiza medição")) -> ()
                n121 = property on="Realiza medição WT230" class="Bool (strict)"("DisabledEnum"=T15."Enabled" ("Disabled")) -> ()  [unwired: 2 in, 2 out]
              }
            }
          }
        }
        n122 = local read "STOP"() -> (w570:bool)
      }
      n123 = call-poly <vilib>:"Write Delimited Spreadsheet.vi"("file path (dialog if empty)"=w118, "1D data"=string[] ["t", "PV [ºC]", "SP [ºC]", "MV[%] "] ("appended array"), "append to file? (new file:F)"=TRUE, "transpose? (no:F)"=FALSE) -> ("new file path (Not A Path if cancelled)"=w119:path)  [unwired: 10 in, 1 out]
      n124 = call-poly <vilib>:"Write Delimited Spreadsheet.vi"("file path (dialog if empty)"=w117, "1D data"=string[] ["t", "PC(E)", "PL(E)", "PC(T)", "PL(T)", "Vel"] ("appended array"), "append to file? (new file:F)"=TRUE, "transpose? (no:F)"=FALSE) -> ("new file path (Not A Path if cancelled)"=w113:path)  [unwired: 10 in, 1 out]
      n125 = call-poly <vilib>:"Write Delimited Spreadsheet.vi"("file path (dialog if empty)"=w112, "1D data"=string[] ["t", "IF", "IR", "VF", "VR"] ("appended array"), "append to file? (new file:F)"=TRUE, "transpose? (no:F)"=FALSE) -> ("new file path (Not A Path if cancelled)"=w108:path)  [unwired: 10 in, 1 out]
      n126 = call-poly <vilib>:"Write Delimited Spreadsheet.vi"("file path (dialog if empty)"=w94, "1D data"=string[] ["t", "PV [ºC]", "SP [ºC]", "MV[A]"] ("appended array"), "append to file? (new file:F)"=TRUE, "transpose? (no:F)"=FALSE) -> ("new file path (Not A Path if cancelled)"=w93:path)  [unwired: 10 in, 1 out]
      n127 = call-poly <vilib>:"Write Delimited Spreadsheet.vi"("file path (dialog if empty)"=w91, "1D data"=string[] ["t", "FP", "PR[W] ", "P_DC[W]", "PU[W]", "PA[W]", "PT [W]", "IP[A]", "I_DC[A]", "IRMS[A]", "I_ACDC[A]", "", ""] ("appended array"), "append to file? (new file:F)"=TRUE, "transpose? (no:F)"=FALSE) -> ("new file path (Not A Path if cancelled)"=w87:path)  [unwired: 10 in, 1 out]
      n128 = call-poly <vilib>:"Write Delimited Spreadsheet.vi"("file path (dialog if empty)"=w103, "1D data"=string[] ["t", "TP1 [ºC]", "TP2 [ºC]", "TP3 [ºC]", "TP5 [ºC]", "TP6 [ºC]", "TP7 [ºC]", "TP8 [ºC]", "TP10 [ºC]", "TP11 [ºC]", "TP12 [ºC]", "TP13 [ºC]", "TP15 [ºC]"] ("appended array"), "append to file? (new file:F)"=TRUE, "transpose? (no:F)"=FALSE) -> ("new file path (Not A Path if cancelled)"=w102:path)  [unwired: 10 in, 1 out]
      n129 = call <vilib>:"High Resolution Relative Seconds.vi"() -> ("relative seconds"=w107:dbl)
      n130 = while {
        tunnel: w87 -> [w282]
        stop <- w270 stop-if-true
        # "Corrente AC + DC RMS"
        # "Corrente AC RMS"
        # "Corrente DC"
        # "Corrente de Pico"
        # "Potência Total"
        # "Potência Aparente"
        # "Potência Real"
        # "Potência DC"
        # "Potência Reativa"
        # "Fator de Potência"
        # "tempo(s):"
        # "Gerando log das Medidas Elétricas da fonte 6812B"
        n131 = local read "PwrMeas"() -> (w255:T9)
        n132 = local read "CurMeas"() -> (w254:T8)
        n133 = Unbundle(w255) -> ("Power Factor"=w253:dbl, "Reactive Power"=w249:dbl, "DC Power"=w252:dbl, "Real Power"=w251:dbl, "Apparent Power"=w247:dbl, "Total Power"=w248:dbl)
        n134 = Unbundle(w254) -> ("Peak Current"=w246:dbl, "DC Current"=w250:dbl, "AC RMS Current"=w245:dbl, "AC + DC RMS Cur"=w244:dbl)
        n135 = Bundle("Reactive Power"=w249, "Apparent Power"=w247, "Total Power"=w248) -> (w242:T12)  [unwired: 1 in]
        n136 = Bundle("Peak Current"=w246, "AC RMS Current"=w245, "AC + DC RMS Cur"=w244) -> (w243:T17)  [unwired: 1 in]
        n137 = local write "ACP_PWR"(w242) -> ()
        n138 = local write "ACP_CUR"(w243) -> ()
        n139 = local read "t"() -> (w277:dbl)
        n140 = Number To Fractional String(number=w277, precision (6)=i16 3) -> (F-format string=w276:string)  [unwired: 2 in]
        n141 = Number To Fractional String(number=w253, precision (6)=i16 3) -> (F-format string=w275:string)  [unwired: 2 in]
        n142 = Number To Fractional String(number=w249, precision (6)=i16 3) -> (F-format string=w272:string)  [unwired: 2 in]
        n143 = Number To Exponential String(number=w252, precision (6)=i16 3) -> (E-format string=w280:string)  [unwired: 2 in]
        n144 = Number To Exponential String(number=w251, precision (6)=i16 3) -> (E-format string=w263:string)  [unwired: 2 in]
        n145 = Number To Exponential String(number=w247, precision (6)=i16 3) -> (E-format string=w262:string)  [unwired: 2 in]
        n146 = Number To Exponential String(number=w248, precision (6)=i16 3) -> (E-format string=w261:string)  [unwired: 2 in]
        n147 = Number To Exponential String(number=w246, precision (6)=i16 3) -> (E-format string=w260:string)  [unwired: 2 in]
        n148 = Number To Exponential String(number=w250, precision (6)=i16 3) -> (E-format string=w259:string)  [unwired: 2 in]
        n149 = Number To Exponential String(number=w245, precision (6)=i16 3) -> (E-format string=w258:string)  [unwired: 2 in]
        n150 = Number To Exponential String(number=w244, precision (6)=i16 3) -> (E-format string=w256:string)  [unwired: 2 in]
        n151 = Build Array(w276, w275, w272, w280, w263, w262, w261, w260, w259, w258, w256) -> (w273:string[])
        n152 = local read "STOP"() -> (w270:bool)
        n153 = call-poly <vilib>:"Write Delimited Spreadsheet.vi"("file path (dialog if empty)"=w282, "1D data"=w273, "append to file? (new file:F)"=TRUE, "transpose? (no:F)"=FALSE) -> ()  [unwired: 10 in, 2 out]
        n154 = Wait (ms)(milliseconds to wait=u32 1000) -> ()  [unwired: 1 out]
      }
      n155 = while {
        tunnel: w93 -> [w389]
        stop <- w374 stop-if-true
        # "tempo(s):"
        # "Saída (PV):"
        # "Referencia (SP):"
        # "sinal de controle (mv):"
        # "Gerando log do Controle do Ensaio Térmico"
        n156 = local read "MV_MF"() -> (w385:sgl)
        n157 = local read "SP_MF"() -> (w378:dbl)
        n158 = local read "PV_MF"() -> (w384:dbl)
        n159 = local read "Time"() -> (w382:dbl)
        n160 = Number To Exponential String(number=w385, precision (6)=i16 3) -> (E-format string=w387:string)  [unwired: 2 in]
        n161 = Number To Fractional String(number=w382, precision (6)=i16 3) -> (F-format string=w381:string)  [unwired: 2 in]
        n162 = Number To Fractional String(number=w384, precision (6)=i16 3) -> (F-format string=w380:string)  [unwired: 2 in]
        n163 = Number To Fractional String(number=w378, precision (6)=i16 3) -> (F-format string=w376:string)  [unwired: 2 in]
        n164 = local read "STOP"() -> (w374:bool)
        n165 = Build Array(w381, w380, w376, w387) -> (w377:string[])
        n166 = call-poly <vilib>:"Write Delimited Spreadsheet.vi"("file path (dialog if empty)"=w389, "1D data"=w377, "append to file? (new file:F)"=TRUE, "transpose? (no:F)"=FALSE) -> ()  [unwired: 10 in, 2 out]
        n167 = Wait (ms)(milliseconds to wait=u32 1000) -> ()  [unwired: 1 out]
      }
      n168 = while {
        tunnel: w119 -> [w737]
        stop <- w722 stop-if-true
        # "tempo(s):"
        # "Saída (PV):"
        # "Referencia (SP):"
        # "sinal de controle (mv):"
        # "Gerando log do Controle de Temperatura da Estufa"
        n169 = local read "Duty Cycle"() -> (w734:sgl)
        n170 = Wait (ms)(milliseconds to wait=u32 1000) -> ()  [unwired: 1 out]
        n171 = local read "SP:"() -> (w727:dbl)
        n172 = local read "PV"() -> (w733:dbl)
        n173 = local read "t"() -> (w731:dbl)
        n174 = Number To Exponential String(number=w734, precision (6)=i16 3) -> (E-format string=w735:string)  [unwired: 2 in]
        n175 = Number To Fractional String(number=w731, precision (6)=i16 3) -> (F-format string=w730:string)  [unwired: 2 in]
        n176 = Number To Fractional String(number=w733, precision (6)=i16 3) -> (F-format string=w729:string)  [unwired: 2 in]
        n177 = Number To Fractional String(number=w727, precision (6)=i16 3) -> (F-format string=w725:string)  [unwired: 2 in]
        n178 = Build Array(w730, w729, w725, w735) -> (w726:string[])
        n179 = local read "STOP"() -> (w722:bool)
        n180 = call-poly <vilib>:"Write Delimited Spreadsheet.vi"("file path (dialog if empty)"=w737, "1D data"=w726, "append to file? (new file:F)"=TRUE, "transpose? (no:F)"=FALSE) -> ()  [unwired: 10 in, 2 out]
      }
      n181 = while {
        tunnel: w108 -> [w543]
        tunnel: w107 -> [w523]
        stop <- w529 stop-if-true
        # "era 200"
        # "Tensão do freio (SP) [V]:"
        # "tempo(s):"
        # "Corrente de saída da fonte [A]:"
        # "Corrente do freio (SP) [A]:"
        # "Tensão de saída da Fonte [V]"
        # "Gerando log dos valores de tensão e corrente enviados ao freio"
        n182 = call <vilib>:"High Resolution Relative Seconds.vi"() -> ("relative seconds"=w524:dbl)
        n183 = Subtract(x=w524, y=w523) -> (x-y=w522:dbl)
        n184 = local write "t"(w522) -> ()
        n185 = local read "Limite de tensão"() -> (w527:dbl)
        n186 = local read "Tensão de saída"() -> (w539:dbl)
        n187 = local read "Limite de corrente"() -> (w532:dbl)
        n188 = local read "Corrente de saída"() -> (w538:dbl)
        n189 = local read "t"() -> (w536:dbl)
        n190 = Number To Exponential String(number=w527, precision (6)=i16 3) -> (E-format string=w525:string)  [unwired: 2 in]
        n191 = Number To Exponential String(number=w539, precision (6)=i16 3) -> (E-format string=w541:string)  [unwired: 2 in]
        n192 = Number To Fractional String(number=w536, precision (6)=i16 3) -> (F-format string=w535:string)  [unwired: 2 in]
        n193 = Number To Fractional String(number=w538, precision (6)=i16 3) -> (F-format string=w534:string)  [unwired: 2 in]
        n194 = Number To Fractional String(number=w532, precision (6)=i16 3) -> (F-format string=w530:string)  [unwired: 2 in]
        n195 = Build Array(w535, w534, w530, w541, w525) -> (w531:string[])
        n196 = local read "STOP"() -> (w529:bool)
        n197 = call-poly <vilib>:"Write Delimited Spreadsheet.vi"("file path (dialog if empty)"=w543, "1D data"=w531, "append to file? (new file:F)"=TRUE, "transpose? (no:F)"=FALSE) -> ()  [unwired: 10 in, 2 out]
        n198 = Wait (ms)(milliseconds to wait=u32 1000) -> ()  [unwired: 1 out]
      }
      n199 = while {
        tunnel: w102 -> [w519]
        stop <- w505 stop-if-true
        # "Termopar Dissipador"
        # "Termopar uC IC601"
        # "Termopar Cap 504"
        # "Termopar Cap C112"
        # "Termopar Indutor L100"
        # "Termopar  IC100"
        # "Termopar Conector"
        # "Termopar Fusivel"
        # "Termopar Cap C006"
        # "tempo(s):"
        # "Termopar Cap C011"
        # "Termopar Cap C009"
        # "Termopar Choke L001"
        # "Gerando log das Temperaturas dos Termopares"
        n200 = local read "TP 3"() -> (w515:dbl)
        n201 = local read "TP 5"() -> (w502:dbl)
        n202 = local read "TP 6"() -> (w501:dbl)
        n203 = local read "TP 7"() -> (w498:dbl)
        n204 = local read "TP 8"() -> (w497:dbl)
        n205 = local read "TP 10"() -> (w494:dbl)
        n206 = local read "TP 11"() -> (w493:dbl)
        n207 = local read "TP 12"() -> (w490:dbl)
        n208 = local read "TP 15"() -> (w487:dbl)
        n209 = local read "TP 1"() -> (w504:dbl)
        n210 = local read "TP 2"() -> (w509:dbl)
        n211 = local read "TP 13"() -> (w489:dbl)
        n212 = local read "t"() -> (w513:dbl)
        n213 = Number To Fractional String(number=w513, precision (6)=i16 3) -> (F-format string=w512:string)  [unwired: 2 in]
        n214 = Number To Fractional String(number=w504, precision (6)=i16 3) -> (F-format string=w511:string)  [unwired: 2 in]
        n215 = Number To Fractional String(number=w509, precision (6)=i16 3) -> (F-format string=w507:string)  [unwired: 2 in]
        n216 = Number To Exponential String(number=w515, precision (6)=i16 3) -> (E-format string=w517:string)  [unwired: 2 in]
        n217 = Number To Exponential String(number=w502, precision (6)=i16 3) -> (E-format string=w486:string)  [unwired: 2 in]
        n218 = Number To Exponential String(number=w501, precision (6)=i16 3) -> (E-format string=w485:string)  [unwired: 2 in]
        n219 = Number To Exponential String(number=w498, precision (6)=i16 3) -> (E-format string=w484:string)  [unwired: 2 in]
        n220 = Number To Exponential String(number=w497, precision (6)=i16 3) -> (E-format string=w483:string)  [unwired: 2 in]
        n221 = Number To Exponential String(number=w494, precision (6)=i16 3) -> (E-format string=w482:string)  [unwired: 2 in]
        n222 = Number To Exponential String(number=w493, precision (6)=i16 3) -> (E-format string=w481:string)  [unwired: 2 in]
        n223 = Number To Exponential String(number=w490, precision (6)=i16 3) -> (E-format string=w480:string)  [unwired: 2 in]
        n224 = Number To Exponential String(number=w489, precision (6)=i16 3) -> (E-format string=w479:string)  [unwired: 2 in]
        n225 = Number To Exponential String(number=w487, precision (6)=i16 3) -> (E-format string=w478:string)  [unwired: 2 in]
        n226 = Build Array(w512, w511, w507, w517, w486, w485, w484, w483, w482, w481, w480, w479, w478) -> (w508:string[])
        n227 = local read "STOP"() -> (w505:bool)
        n228 = call-poly <vilib>:"Write Delimited Spreadsheet.vi"("file path (dialog if empty)"=w519, "1D data"=w508, "append to file? (new file:F)"=TRUE, "transpose? (no:F)"=FALSE) -> ()  [unwired: 10 in, 2 out]
        n229 = Wait (ms)(milliseconds to wait=u32 1000) -> ()  [unwired: 1 out]
      }
      n230 = while {
        tunnel: w113 -> [w567]
        stop <- w553 stop-if-true
        # "era 200"
        # "SP de velocidade do motor:"
        # "Pot. lida total"
        # "tempo(s):"
        # "Pot. calculada na entrada do IF:"
        # "Pot. lida na entrada do IF:"
        # "Pot. calculada total"
        # "Gerando log das potências medidas  do IF feitas pelo  Wattímetro"
        n231 = local read "Velocidade (RPM)"() -> (w549:u16)
        n232 = local read "PL(T)"() -> (w552:dbl)
        n233 = local read "PC(T)"() -> (w563:dbl)
        n234 = local read "PL(E)"() -> (w556:dbl)
        n235 = local read "PC(E)"() -> (w562:dbl)
        n236 = local read "t"() -> (w560:dbl)
        n237 = Number To Exponential String(number=w552, precision (6)=i16 3) -> (E-format string=w550:string)  [unwired: 2 in]
        n238 = Number To Exponential String(number=w563, precision (6)=i16 3) -> (E-format string=w565:string)  [unwired: 2 in]
        n239 = Number To Exponential String(number=w549, precision (6)=i16 3) -> (E-format string=w546:string)  [unwired: 2 in]
        n240 = Number To Fractional String(number=w560, precision (6)=i16 3) -> (F-format string=w559:string)  [unwired: 2 in]
        n241 = Number To Fractional String(number=w562, precision (6)=i16 3) -> (F-format string=w558:string)  [unwired: 2 in]
        n242 = Number To Fractional String(number=w556, precision (6)=i16 3) -> (F-format string=w554:string)  [unwired: 2 in]
        n243 = Build Array(w559, w558, w554, w565, w550, w546) -> (w555:string[])
        n244 = local read "STOP"() -> (w553:bool)
        n245 = call-poly <vilib>:"Write Delimited Spreadsheet.vi"("file path (dialog if empty)"=w567, "1D data"=w555, "append to file? (new file:F)"=TRUE, "transpose? (no:F)"=FALSE) -> ()  [unwired: 10 in, 2 out]
        n246 = Wait (ms)(milliseconds to wait=u32 1000) -> ()  [unwired: 1 out]
      }
      n247 = while {
        stop <- w661 stop-if-true
        # "Malha de controle de Temperatura da Estufa  - PI"
        n248 = local read "PV"() -> (w665:dbl)
        n249 = Bundle("PV"=w665, "SP:"="SP:") -> (→"Process variable and Setpoint":cluster{"PV":dbl, "SP:":dbl})  [unwired: 1 in]
        n250 = call-poly <vilib>:"PID.vi"("output range"=cluster{"output high":dbl, "output low":dbl} {"output high"=99.9, "output low"=0.01}, "PID gains"="PID gains", "process variable"=w665, "setpoint"="SP:") -> ("output"=w660:dbl)  [unwired: 6 in, 1 out]
        "MV" <- w660
        n251 = local write "Duty Cycle"(w660) -> ()
        n252 = Multiply(x="Ts", y=u32 1000 ("unsigned 32bit integer")) -> (x*y=w659:dbl)
        n253 = local read "STOP"() -> (w661:bool)
        n254 = Wait Until Next ms Multiple(millisecond multiple=w659) -> ()  [unwired: 1 out]
      }
      n255 = while {
        stop <- w338 stop-if-true
        # "Ensaio térmico automatizado"
        n256 = Not(x="Manual") -> (.not. x?=w337:bool)
        n257 = case shown="True" w337 {
          frame False {
            n258 = local write "Automatic"(FALSE ("Automatic")) -> ()
          }
          frame True {
            # "TP5 = valor limite?"
            # "T_estufa = SP?"
            n259 = local read "SP:"() -> (w348:dbl)
            n260 = local read "PV_MF"() -> (w341:dbl)
            n261 = local read "SP_MF"() -> (w342:dbl)
            n262 = local read "STOP"() -> (w352:bool)
            n263 = local read "PV"() -> (w347:dbl)
            n264 = call "noslimites.vi"("lim"=0.1, "PVx"=w342, "SPx:"=w341) -> ("Está dentro dos limites?"=w344:bool)  [unwired: 8 in]
            n265 = call "noslimites.vi"("lim"=1.0, "PVx"=w347, "SPx:"=w348) -> ("Está dentro dos limites?"=w345:bool)  [unwired: 8 in]
            n266 = Not(x=w344) -> (.not. x?=w340:bool)
            n267 = Not(x=w352) -> (.not. x?=w350:bool)
            n268 = And(x=w345, y=w340) -> (x .and. y?=w351:bool)
            n269 = And(x=w351, y=w350) -> (x .and. y?=w349:bool)
            n270 = case shown="False" w349 {
              frame False {
                w355 = FALSE ("data")
                w356 = refnum<k21> "resfriamento_freio"  # DAQmx Task Name
                # "Desliga freio e o resfriamento do freio, para motor \ne desliga controle automatico"
                n271 = local write "Automatic"(FALSE ("Liga Fonte")) -> ()
                n272 = local read "Parâmetros serial"() -> (w359:T4)
                n273 = call <instrlib>:"GENie Config Output On-Off.vi"("Output ON"=w355, "VISA"=refnum<visa-resource-name> "Lambda" ("VISA name")) -> ()  [unwired: 8 in, 2 out]
                n274 = call "Serial_control.vi"("Enviar número"=u16 0, "Função"=T13."Set Speed", "comm cluster"=w359) -> ("translated message"=w361:string, "read buffer"=w360:string)  [unwired: 2 in, 2 out]
                n275 = call-poly <vilib>:"DAQmx Write.vi"("task/channels in"=w356, "data"=w355) -> ()  [unwired: 11 in, 3 out]
                n276 = local write "Resposta"(w360) -> ()
                n277 = local write "Tradução"(w361) -> ()
              }
              frame True {
                n278 = flat-sequence {
                  frame #0 {
                    # "Liga o motor a 3000 RPM"
                    n279 = local read "Parâmetros serial"() -> (w363:T4)
                    n280 = local write "Parar motor"(FALSE ("Parar motor")) -> ()
                    n281 = call "Serial_control.vi"("Enviar número"=u16 3000, "Função"=T13."Set Speed", "comm cluster"=w363) -> ("translated message"=w366:string, "read buffer"=w365:string)  [unwired: 2 in, 2 out]
                    n282 = local write "Resposta"(w365) -> ()
                    n283 = local write "Tradução"(w366) -> ()
                  }
                  frame #1 {
                    w368 = u32 4000  # Interval
                    # "Espera atingir a vel"
                    n284 = Wait (ms)(milliseconds to wait=w368) -> ()  [unwired: 1 out]
                  }
                  frame #2 {
                    w369 = TRUE ("data")
                    w371 = refnum<k21> "resfriamento_freio"  # DAQmx Task Name
                    # "Liga o freio e o resfriamento do freio"
                    n285 = call <instrlib>:"GENie Config Output On-Off.vi"("Output ON"=w369, "VISA"=refnum<visa-resource-name> "Lambda" ("VISA name")) -> ()  [unwired: 8 in, 2 out]
                    n286 = call-poly <vilib>:"DAQmx Write.vi"("task/channels in"=w371, "data"=w369) -> ()  [unwired: 11 in, 3 out]
                  }
                  frame #3 {
                    w372 = u32 3000  # Interval
                    # "Espera o motor acomodar"
                    n287 = Wait (ms)(milliseconds to wait=w372) -> ()  [unwired: 1 out]
                  }
                  frame #4 {
                    # "Liga controle auto"
                    n288 = local write "Automatic"(TRUE ("Liga Fonte")) -> ()
                  }
                }
              }
            }
          }
        }
        n289 = local read "STOP"() -> (w338:bool)
      }
      n290 = call <vilib>:"High Resolution Relative Seconds.vi"() -> ("relative seconds"=w100:dbl)
      n291 = call <instrlib>:"Close.vi"("error in (no error)"=w85, "VISA resource name"=w86) -> ("error out"=w79:errorcluster)  [unwired: 9 in]
      n292 = call <vilib>:"Simple Error Handler.vi"("error in (no error)"=w79) -> ()  [unwired: 4 in, 5 out]
      n293 = while {
        tunnel: [w459] -> w101
        tunnel: w100 -> [w400]
        tunnel: [w399] -> w99
        tunnel: w98 -> [w392]
        i -> [w398]
        stop <- w462 stop-if-true
        # "temp. do termopar a ser controlada pelo controlador Ens. Ter. em MF"
        # "PT100"
        # "DAQ Temperatura Termopares do  IF e dos PT100 de Temperatura  do Forno e do Dinamômetro"
        n294 = call <vilib>:"High Resolution Relative Seconds.vi"() -> ("relative seconds"=w416:dbl)
        n295 = call <vilib>:"High Resolution Polling Wait.vi"("seconds to wait"=1.0) -> ()  [unwired: 10 in, 1 out]
        n296 = Subtract(x=w416, y=w400) -> (x-y=w412:dbl)
        n297 = local write "Time"(w412) -> ()
        n298 = call <instrlib>:"EZ Temperature.vi"("VISA Resource Name"=w392, "Scan List (empty)"="301,302,303,305,306,307,308,310,311,312,313,315", "Transducer Type (4:Def-Last)"=T14."Thermocouple") -> ("VISA Resource Name Out"=w459:refnum<visa-resource-name>, "Output Array"=w465:dbl[])  [unwired: 10 in, 1 out]
        n299 = Index Array(array=w465, index #1=0 ("index"), index #2=1 ("index"), index #3=2 ("index"), index #4=3 ("index"), index #5=4 ("index"), index #6=5 ("index"), index #7=6 ("index"), index #8=7 ("index"), index #9=8 ("index"), index #10=9 ("index"), index #11=10 ("index"), index #12=11 ("index")) -> (element #1=w396:dbl, element #3=w436:dbl, element #4=w397:dbl, element #5=w435:dbl, element #6=w434:dbl, element #7=w433:dbl, element #8=w432:dbl, element #9=w431:dbl, element #10=w430:dbl, element #11=w429:dbl, element #12=w428:dbl)  [unwired: 1 out]
        n300 = local write "TP 1"(w396) -> ()
        n301 = local write "TP 3"(w436) -> ()
        n302 = local write "TP 5"(w397) -> ()
        n303 = local write "TP 6"(w435) -> ()
        n304 = local write "TP 7"(w434) -> ()
        n305 = local write "TP 8"(w433) -> ()
        n306 = local write "TP 10"(w432) -> ()
        n307 = local write "TP 11"(w431) -> ()
        n308 = local write "TP 12"(w430) -> ()
        n309 = local write "TP 13"(w429) -> ()
        n310 = local write "TP 15"(w428) -> ()
        n311 = Bundle(w396, "index"=70) -> (→"G. TP 1":cluster{dbl, "index":i32})  [unwired: 1 in]
        n312 = Bundle(w397, "index"=68) -> (→"G. TP 5":cluster{dbl, "index":i32})  [unwired: 1 in]
        n313 = Bundle(w431, "index"=65) -> (→"G. TP 11":cluster{dbl, "index":i32})  [unwired: 1 in]
        n314 = Bundle(w430, "index"=73) -> (→"G. TP 12":cluster{dbl, "index":i32})  [unwired: 1 in]
        n315 = Bundle(w429, "index"=74) -> (→"G. TP 13":cluster{dbl, "index":i32})  [unwired: 1 in]
        n316 = Bundle(w428, "index"=80) -> (→"G. TP 15":cluster{dbl, "index":i32})  [unwired: 1 in]
        n317 = Bundle(w436, "index"=68) -> (→"G. TP 3":cluster{dbl, "index":i32})  [unwired: 1 in]
        n318 = Bundle(w435, "index"=69) -> (→"G. TP 6":cluster{dbl, "index":i32})  [unwired: 1 in]
        n319 = Bundle(w434, "index"=63) -> (→"G. TP 7":cluster{dbl, "index":i32})  [unwired: 1 in]
        n320 = Bundle(w433, "index"=76) -> (→"G. TP 8":cluster{dbl, "index":i32})  [unwired: 1 in]
        n321 = Bundle(w432, "index"=78) -> (→"G. TP 10":cluster{dbl, "index":i32})  [unwired: 1 in]
        n322 = Add(x=w396, y=0.015) -> (x+y=w395:dbl)
        n323 = local write "TP 2"(w395) -> ()
        n324 = Bundle(w395, "index"=70) -> (→"G. TP 2":cluster{dbl, "index":i32})  [unwired: 1 in]
        n325 = local write "PV_MF"(w396) -> ()
        n326 = call <instrlib>:"EZ Temperature.vi"("VISA Resource Name"=w392, "Scan List (empty)"="101,102,103, 104, 105, 106, 304,309", "Transducer Type (4:Def-Last)"=T14."4-Wire RTD") -> ("VISA Resource Name Out"=w399:refnum<visa-resource-name>, "Output Array"=w413:dbl[])  [unwired: 10 in, 1 out]
        n327 = Index Array(array=w413, index #1=0 ("index"), index #2=1 ("index"), index #3=2 ("index"), index #4=3 ("index"), index #5=4 ("index"), index #6=5 ("index"), index #7=6 ("index"), index #8=7 ("index")) -> (element #1=w419:dbl, element #2=w420:dbl, element #3=w421:dbl, element #4=w422:dbl, element #5=w423:dbl, element #6=w424:dbl, element #7=w425:dbl, element #8=w426:dbl)
        n328 = Add(x=w425, y=w426) -> (x+y=w414:dbl)
        n329 = Bundle(w419, w420, w421, w422, w423, w424) -> (→"Chart Temperatura":cluster{dbl, dbl, dbl, dbl, dbl, dbl})  [unwired: 1 in]
        n330 = Bundle(w419, w420, w421, w422, w423, w424) -> (→"temperature num cluster":cluster{dbl, dbl, dbl, dbl, dbl, dbl})  [unwired: 1 in]
        n331 = local write "Temperature CH4 [degC]"(w425) -> ()
        n332 = local write "Temperature CH9 [degC]"(w426) -> ()
        n333 = Divide(x=w414, y=2.0) -> (x/y=w415:dbl)
        n334 = local read "STOP"() -> (w462:bool)
        n335 = local write "PV"(w415) -> ()
        "Iteration" <- w398
      }
      n336 = while {
        stop <- w669 stop-if-true
        # "PWM Generator"
        n337 = local read "Estufa_ON"() -> (w670:bool)
        n338 = case shown="True" w670 {
          frame False {
            n339 = Wait (ms)(milliseconds to wait=u32 100) -> ()  [unwired: 1 out]
          }
          frame True {
            w678 = T18 0 items=["no dialog", "OK message", "continue or stop message", "OK message + warnings", "continue/stop + warnings"] ("type of dialog (OK msg:1)")
            w689 = 10123 items=["Finite Samples"=10178, "Continuous Samples"=10123, "Hardware Timed Single Point"=12522]  # Sample Mode
            n340 = local read "Duty Cycle"() -> (w673:sgl)
            n341 = Divide(x=w673, y=100.0) -> (x/y=w672:dbl)
            n342 = local read "Frequency"() -> (w675:dbl)
            n343 = call-poly <vilib>:"DAQmx Create Virtual Channel.vi"("frequency"=w675, "duty cycle"=w672, "counter"=tag "Dev1/ctr3" ("Counter")) -> ("task out"=w692:refnum<k21>, "error out"=w691:errorcluster)  [unwired: 11 in]
            n344 = property class="DAQmx Channel"(reference=w692, error in=w691, "CO.Pulse.Term"=tag "/Dev1/PFI15" ("Output Terminal")) -> (reference out=w688:refnum<k21>, error out=w687:errorcluster)
            n345 = call-poly <vilib>:"DAQmx Timing.vi"("task/channels in"=w688, "sample mode"=w689, "error in"=w687) -> ("task out"=w686:refnum<k21>, "error out"=w685:errorcluster)  [unwired: 11 in]
            n346 = call <vilib>:"DAQmx Start Task.vi"("task/channels in"=w686, "error in"=w685) -> ("task out"=w684:refnum<k21>, "error out"=w683:errorcluster)  [unwired: 12 in]
            n347 = while {
              tunnel: w684 -> [w703]
              tunnel: w683 -> [w701]
              tunnel: [w712] -> w680
              tunnel: [w713] -> w681
              tunnel: [FALSE ("Liga aquecedor")] -> w677
              tunnel: w672 -> [w699]
              tunnel: w675 -> [w697]
              stop <- w706 stop-if-true
              # "era F"
              n348 = local read "Duty Cycle"() -> (w696:sgl)
              n349 = Wait Until Next ms Multiple(millisecond multiple=u32 10) -> ()  [unwired: 1 out]
              n350 = Divide(x=w696, y=100.0) -> (x/y=w694:dbl)
              n351 = Not Equal?(x=w699, y=w694) -> (x != y?=w698:bool)
              n352 = case shown="True" w698 {
                tunnel: [w715 w718] -> w702
                tunnel: w703 -> [w715 w719]
                tunnel: [w714 w720] -> w700
                tunnel: w701 -> [w714 w721]
                tunnel: w694 -> [_ w717]
                tunnel: w697 -> [_ w716]
                frame False {
                }
                frame True {
                  n353 = call-poly <vilib>:"DAQmx Write.vi"("task/channels in"=w719, "frequency"=w716, "duty cycle"=w717, "error in"=w721) -> ("task out"=w718:refnum<k21>, "error out"=w720:errorcluster)  [unwired: 9 in, 1 out]
                }
              }
              n354 = call <vilib>:"DAQmx Is Task Done.vi"("task/channels in"=w702, "error in"=w700) -> ("task out"=w713:refnum<k21>, "error out"=w712:errorcluster)  [unwired: 11 in, 1 out]
              n355 = local read "Estufa_ON"() -> (w709:bool)
              n356 = Unbundle By Name(w712) -> ("status"=w711:bool)
              n357 = Not(x=w709) -> (.not. x?=w707:bool)
              n358 = local read "STOP"() -> (w704:bool)
              n359 = Or(x=w711, y=w707) -> (x .or. y?=w705:bool)
              n360 = Or(x=w705, y=w704) -> (x .or. y?=w706:bool)
            }
            n361 = call <vilib>:"DAQmx Stop Task.vi"("task/channels in"=w681, "error in"=w680) -> ("task out"=w676:refnum<k21>, "error out"=w682:errorcluster)  [unwired: 12 in]
            n362 = local write "Estufa_ON"(w677) -> ()
            n363 = call <vilib>:"DAQmx Clear Task.vi"("task in"=w676, "error in"=w682) -> ("error out"=w679:errorcluster)  [unwired: 13 in]
            n364 = call <vilib>:"Simple Error Handler.vi"("error code (no error:0)"=w678, "error in (no error)"=w679) -> ()  [unwired: 3 in, 5 out]
          }
        }
        n365 = local read "STOP"() -> (w669:bool)
      }
      n366 = while {
        tunnel: w92 -> [w286]
        stop <- w285 stop-if-true
        # "Aquisição - Fonte DC"
        n367 = call <instrlib>:"GENie Meas Output Voltage.vi"("VISA"=w286) -> ("Output Voltage"=→"Tensão de saída":dbl, "VISA out"=w289:refnum<visa-resource-name>)  [unwired: 8 in, 1 out]
        n368 = Wait (ms)(milliseconds to wait=u32 200) -> ()  [unwired: 1 out]
        n369 = call <instrlib>:"GENie Meas Output Current.vi"("VISA"=w289) -> ("Output Current"=→"Corrente de saída":dbl)  [unwired: 8 in, 2 out]
        n370 = local read "STOP"() -> (w285:bool)
      }
      n371 = while {
        tunnel: w92 -> [w291]
        stop <- w292 stop-if-true
        # "Tratador de eventos manuais controlados pela IHM"
        n372 = event shown="[1] \"STOP\": Value Change" {
          selector: _ -> [_ _ _ _ _ _]
          dyn-events: _ -> [_ _ _ _ _ _]
          timeout: _ -> [_ _ _ _ _ _]
          tunnel: w291 -> [_ w300 _ _ w323 w329]
          tunnel: [_ w301 _ _ _ _] -> w292
          event "Enviar velocidade": Value Change {
            n373 = event-data() -> ("OldVal"=w298:bool)  [unwired: 1 in, 5 out]
            n374 = local read "Parâmetros serial"() -> (w297:T4)
            n375 = local write "Enviar velocidade"(w298) -> ()
            n376 = call "Serial_control.vi"("Enviar número"="Velocidade (RPM)", "Função"=T13."Set Speed", "comm cluster"=w297) -> ("translated message"=w294:string, "read buffer"=w295:string)  [unwired: 2 in, 2 out]
            n377 = local write "Resposta"(w295) -> ()
            n378 = local write "Tradução"(w294) -> ()
          }
          event "STOP": Value Change {
            w299 = FALSE ("Output ON")
            # "desliga fonte de corrente"
            # "para o motor"
            n379 = event-data() -> ("NewVal"=w301:bool)  [unwired: 1 in, 5 out]
            n380 = local read "Parâmetros serial"() -> (w306:T4)
            n381 = call <instrlib>:"GENie Config Output On-Off.vi"("Output ON"=w299, "VISA"=w300) -> ()  [unwired: 8 in, 2 out]
            n382 = local write "Liga Fonte"(w299) -> ()
            n383 = local write "Automatic"(w299) -> ()
            n384 = call "Serial_control.vi"("Enviar número"=u16 0, "Função"=T13."Set Speed", "comm cluster"=w306) -> ("translated message"=w304:string, "read buffer"=w305:string)  [unwired: 2 in, 2 out]
            n385 = local write "Resposta"(w305) -> ()
            n386 = local write "Tradução"(w304) -> ()
          }
          event "Parar motor": Value Change {
            n387 = event-data() -> ("OldVal"=w309:bool)  [unwired: 1 in, 5 out]
            n388 = local write "Parar motor"(w309) -> ()
            n389 = local read "Parâmetros serial"() -> (w312:T4)
            n390 = call "Serial_control.vi"("Enviar número"=u16 0, "Função"=T13."Set Speed", "comm cluster"=w312) -> ("translated message"=w307:string, "read buffer"=w308:string)  [unwired: 2 in, 2 out]
            n391 = local write "Resposta"(w308) -> ()
            n392 = local write "Tradução"(w307) -> ()
          }
          event "Envia mensagem": Value Change {
            n393 = event-data() -> ("OldVal"=w318:bool)  [unwired: 1 in, 5 out]
            n394 = local write "Envia mensagem"(w318) -> ()
            n395 = local read "Parâmetros serial"() -> (w317:T4)
            n396 = call "Serial_control.vi"("Message"="Mensagem", "Função"=T13."Send Static Message", "comm cluster"=w317) -> ("translated message"=w315:string, "read buffer"=w314:string)  [unwired: 2 in, 2 out]
            n397 = local write "Resposta"(w314) -> ()
            n398 = local write "Tradução"(w315) -> ()
          }
          event "Seta carga": Value Change {
            n399 = event-data() -> ("NewVal"=w319:bool)  [unwired: 1 in, 5 out]
            n400 = local read "Automatic"() -> (w320:bool)
            n401 = local write "Seta carga"(w319) -> ()
            n402 = case shown="True" w320 {
              tunnel: ["Limite de corrente" w326] -> w321
              frame False {
              }
              frame True {
                n403 = local read "MV_MF"() -> (w326:sgl)
              }
            }
            n404 = call <instrlib>:"GENie Config Current Limit.vi"("Current Limit"=w321, "VISA"=w323) -> ("VISA out"=w322:refnum<visa-resource-name>)  [unwired: 8 in, 1 out]
            n405 = call <instrlib>:"GENie Config Voltage Limit.vi"("Volt Limit"="Limite de tensão", "VISA"=w322) -> ()  [unwired: 8 in, 2 out]
          }
          event "Liga Fonte": Value Change {
            w328 = refnum<k21> "resfriamento_freio"  # DAQmx Task Name
            n406 = event-data() -> ("NewVal"=w327:bool)  [unwired: 1 in, 5 out]
            n407 = call <instrlib>:"GENie Config Output On-Off.vi"("Output ON"=w327, "VISA"=w329) -> ()  [unwired: 8 in, 2 out]
            n408 = call-poly <vilib>:"DAQmx Write.vi"("task/channels in"=w328, "data"=w327) -> ()  [unwired: 11 in, 3 out]
          }
        }
      }
      n409 = while {
        stop <- w232 stop-if-true
        # "Malha de controle do Ensaio Térmico"
        n410 = local read "Manual"() -> (w228:bool)
        n411 = local read "Automatic"() -> (w230:bool)
        n412 = Not(x=w228) -> (.not. x?=w229:bool)
        n413 = And(x=w230, y=w229) -> (x .and. y?=w231:bool)
        n414 = case shown="True" w231 {
          frame False {
          }
          frame True {
            n415 = local read "PV_MF"() -> (w238:dbl)
            n416 = Bundle("PV_MF"=w238, "SP_MF"="SP_MF") -> (→"Grafico MF ENS":cluster{"PV_MF":dbl, "SP_MF":dbl})  [unwired: 1 in]
            n417 = call-poly <vilib>:"PID.vi"("output range"=cluster{"output high":dbl, "output low":dbl} {"output high"=0.31, "output low"=0.0}, "PID gains"="PID gains MF", "process variable"=w238, "setpoint"="SP_MF") -> ("output"=w233:dbl)  [unwired: 6 in, 1 out]
            "MV_I" <- w233
            n418 = Multiply(x="Ts MF", y=u32 1000 ("unsigned 32bit integer")) -> (x*y=w234:dbl)
            n419 = local write "MV_MF"(w233) -> ()
            n420 = Wait Until Next ms Multiple(millisecond multiple=w234) -> ()  [unwired: 1 out]
          }
        }
        n421 = local read "STOP"() -> (w232:bool)
      }
      n422 = while {
        stop <- w330 stop-if-true
        # "Enviando sinal de controle (corrente) para o freio de histerese continuamente"
        n423 = local read "Automatic"() -> (w331:bool)
        n424 = case shown="True" w331 {
          frame False {
          }
          frame True {
            n425 = flat-sequence {
              frame #0 {
                n426 = local write "Seta carga"(FALSE ("Seta carga")) -> ()
              }
              frame #1 {
                n427 = local read "MV_MF"() -> (w334:sgl)
                n428 = call <instrlib>:"GENie Config Current Limit.vi"("Current Limit"=w334, "VISA"=refnum<visa-resource-name> "Lambda" ("VISA name")) -> ()  [unwired: 8 in, 2 out]
              }
              frame #2 {
                n429 = local write "Seta carga"(TRUE ("Seta carga")) -> ()
              }
            }
          }
        }
        n430 = local read "STOP"() -> (w330:bool)
      }
      n431 = call <instrlib>:"Close.vi"("VISA Resource Name"=w101) -> ()  [unwired: 14 in, 1 out]
      n432 = call <instrlib>:"Close.vi"("VISA Resource Name"=w99) -> ()  [unwired: 14 in, 1 out]
    }
    frame #2 {
      n433 = local write "STOP"(FALSE ("STOP")) -> ()
    }
  }
